vi "自动搜寻串口.vi"() -> (6 "找到的串口":string[](array[string]), 7 "找到的数量":dbl, 8 "有错误?":bool)   [LabVIEW 2018]
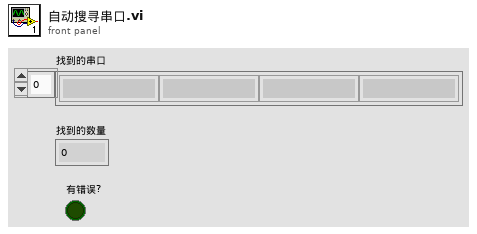
[diagram p1: front panel]
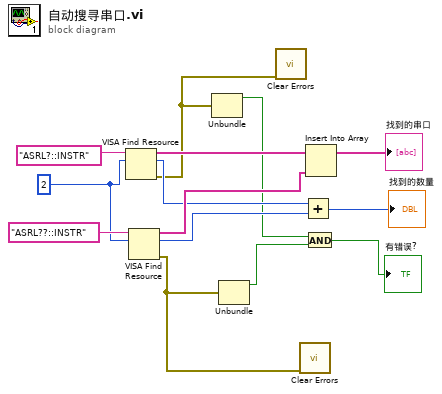
[diagram p0: block diagram]
diagram:
  w10 = 2
  n1 = VISA Find Resource(10:w10, 11:"ASRL?::INSTR") -> (0:w3:errorcluster, 2:w9:u32, 3:w12:string[])  [unwired: 1 in]
  n2 = VISA Find Resource(10:w10, 11:"ASRL??::INSTR") -> (0:w4:errorcluster, 2:w8:u32, 3:w11:string[])  [unwired: 1 in]
  n3 = Unbundle(w3) -> ("status"=w1:bool)  [unwired: 2 out]
  n4 = Unbundle(w4) -> ("status"=w2:bool)  [unwired: 2 out]
  n5 = call <vilib>:"Clear Errors.vi"("error in (no error)"=w3) -> ()  [unwired: 5 in, 2 out]
  n6 = call <vilib>:"Clear Errors.vi"("error in (no error)"=w4) -> ()  [unwired: 5 in, 2 out]
  n7 = Add(x=w9, y=w8) -> (x+y=→"找到的数量":u32)
  n8 = And(x=w1, y=w2) -> (x .and. y?=→"有错误?":bool)
  n9 = Insert Into Array(array=w12, new element=w11) -> (→"找到的串口":string[])  [unwired: 1 in]
